vi "Register gRPC Methods.vi"(8 "error in (no error)":errorcluster, 11 "Template Server in":refnum<class "HVC9.lvclass">) -> (0 "error out":errorcluster, 3 "Template Server out":refnum<class "HVC9.lvclass">)   [LabVIEW 2019, in "HVC9.lvlib" / "HVC9.lvclass"]
uses:
  HVC9.lvclass
  typeDefs/Server Internal UEs.ctl
  typeDefs/Server Internal Message.ctl
  typeDefs/Server gRPC UEs.ctl
  gRPC lvSupport/Server API/typeDefs/gRPCId Cluster.ctl
  gRPC lvSupport/Server API/typeDefs/grpcId.ctl
  HVC9.lvclass/HVC9.ctl
  gRPC lvSupport/gprc-lvsupport.lvlib
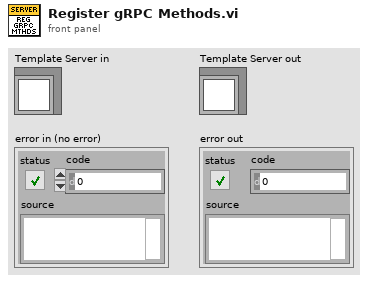
[diagram p1: front panel]
types:
  T1 = typedef "HVC9.lvlib/HVC9.lvclass/Server gRPC UEs.ctl" = cluster{"Invoke gRPC UE":refnum<user-event>, "Query gRPC UE":refnum<user-event>, "Register gRPC UE":refnum<user-event>, "OpenNI2564ASession gRPC UE":refnum<user-event>, "CloseNI2564AChannel gRPC UE":refnum<user-event>, "OpenNI2564AChannel gRPC UE":refnum<user-event>, "DisconnectAllNI2564AChannels gRPC UE":refnum<user-event>, "CloseNI2564ASession gRPC UE":refnum<user-event>, "ResetNI2564A gRPC UE":refnum<user-event>, "OpenNI2564BSession gRPC UE":refnum<user-event>, "CloseNI2564BChannel gRPC UE":refnum<user-event>, "OpenNI2564BChannel gRPC UE":refnum<user-event>, "DisconnectAllNI2564BChannels gRPC UE":refnum<user-event>, "CloseNI2564BSession gRPC UE":refnum<user-event>, "ResetNI2564B gRPC UE":refnum<user-event>}
  T2 = typedef "HVC9.lvlib/HVC9.lvclass/Server Internal UEs.ctl" = cluster{"Invoke Internal UE":refnum<user-event>, "Query Internal UE":refnum<user-event>, "Register Internal UE":refnum<user-event>, "OpenNI2564ASession Internal UE":refnum<user-event>, "CloseNI2564AChannel Internal UE":refnum<user-event>, "OpenNI2564AChannel Internal UE":refnum<user-event>, "DisconnectAllNI2564AChannels Internal UE":refnum<user-event>, "CloseNI2564ASession Internal UE":refnum<user-event>, "ResetNI2564A Internal UE":refnum<user-event>, "OpenNI2564BSession Internal UE":refnum<user-event>, "CloseNI2564BChannel Internal UE":refnum<user-event>, "OpenNI2564BChannel Internal UE":refnum<user-event>, "DisconnectAllNI2564BChannels Internal UE":refnum<user-event>, "CloseNI2564BSession Internal UE":refnum<user-event>, "ResetNI2564B Internal UE":refnum<user-event>}
  T3 = typedef "HVC9.lvlib/gprc-lvsupport.lvlib/grpcId.ctl" = u64
  T4 = typedef "HVC9.lvlib/HVC9.lvclass/Server Internal Message UE.ctl" = refnum<user-event>
  T5 = typedef "HVC9.lvlib/gprc-lvsupport.lvlib/gRPCId Cluster UE.ctl" = refnum<user-event>
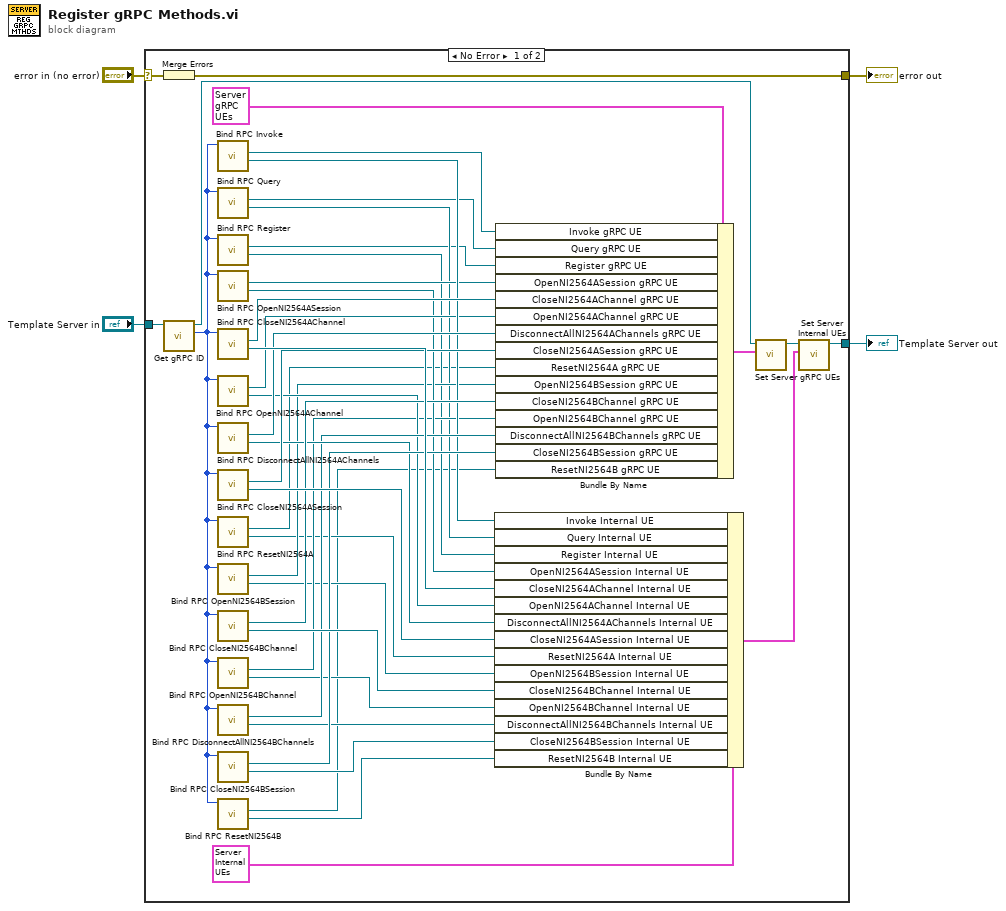
[diagram p0: block diagram]
diagram:
  n1 = case shown="No Error" "error in (no error)" {
    selector: "error in (no error)" -> [w36 w46]
    tunnel: "Template Server in" -> [w44 w47]
    tunnel: [w43 w46] -> w3
    tunnel: [w42 w47] -> w2
    frame No Error {
      n2 = Merge Errors(w36) -> (w43:errorcluster)
      n3 = call "Get gRPC ID.vi"("OOP Server in"=w44) -> ("gRPC ID"=w35:T3, "OOP Server out"=w45:refnum<class "HVC9.lvclass">)  [unwired: 9 in]
      n4 = call "Bind RPC Invoke.vi"("gRPCid server in"=w35) -> ("Invoke Internal UE"=w22:T4, "Invoke gRPC UE"=w21:T5)  [unwired: 7 in, 2 out]
      n5 = call "Bind RPC Query.vi"("gRPCid server in"=w35) -> ("Query Internal UE"=w12:T4, "Query gRPC UE"=w11:T5)  [unwired: 7 in, 2 out]
      n6 = call "Bind RPC Register.vi"("gRPCid server in"=w35) -> ("Register Internal UE"=w10:T4, "Register gRPC UE"=w9:T5)  [unwired: 7 in, 2 out]
      n7 = call "Bind RPC OpenNI2564ASession.vi"("gRPCid server in"=w35) -> ("OpenNI2564ASession Internal UE"=w18:T4, "OpenNI2564ASession gRPC UE"=w17:T5)  [unwired: 7 in, 2 out]
      n8 = call "Bind RPC CloseNI2564AChannel.vi"("gRPCid server in"=w35) -> ("CloseNI2564AChannel Internal UE"=w34:T4, "CloseNI2564AChannel gRPC UE"=w33:T5)  [unwired: 7 in, 2 out]
      n9 = call "Bind RPC OpenNI2564AChannel.vi"("gRPCid server in"=w35) -> ("OpenNI2564AChannel Internal UE"=w20:T4, "OpenNI2564AChannel gRPC UE"=w19:T5)  [unwired: 7 in, 2 out]
      n10 = call "Bind RPC DisconnectAllNI2564AChannels.vi"("gRPCid server in"=w35) -> ("DisconnectAllNI2564AChannels Internal UE"=w26:T4, "DisconnectAllNI2564AChannels gRPC UE"=w25:T5)  [unwired: 7 in, 2 out]
      n11 = call "Bind RPC CloseNI2564ASession.vi"("gRPCid server in"=w35) -> ("CloseNI2564ASession Internal UE"=w32:T4, "CloseNI2564ASession gRPC UE"=w31:T5)  [unwired: 7 in, 2 out]
      n12 = call "Bind RPC ResetNI2564A.vi"("gRPCid server in"=w35) -> ("ResetNI2564A Internal UE"=w8:T4, "ResetNI2564A gRPC UE"=w7:T5)  [unwired: 7 in, 2 out]
      n13 = call "Bind RPC OpenNI2564BSession.vi"("gRPCid server in"=w35) -> ("OpenNI2564BSession Internal UE"=w14:T4, "OpenNI2564BSession gRPC UE"=w13:T5)  [unwired: 7 in, 2 out]
      n14 = call "Bind RPC CloseNI2564BChannel.vi"("gRPCid server in"=w35) -> ("CloseNI2564BChannel Internal UE"=w30:T4, "CloseNI2564BChannel gRPC UE"=w29:T5)  [unwired: 7 in, 2 out]
      n15 = call "Bind RPC OpenNI2564BChannel.vi"("gRPCid server in"=w35) -> ("OpenNI2564BChannel Internal UE"=w16:T4, "OpenNI2564BChannel gRPC UE"=w15:T5)  [unwired: 7 in, 2 out]
      n16 = call "Bind RPC DisconnectAllNI2564BChannels.vi"("gRPCid server in"=w35) -> ("DisconnectAllNI2564BChannels Internal UE"=w24:T4, "DisconnectAllNI2564BChannels gRPC UE"=w23:T5)  [unwired: 7 in, 2 out]
      n17 = call "Bind RPC CloseNI2564BSession.vi"("gRPCid server in"=w35) -> ("CloseNI2564BSession Internal UE"=w28:T4, "CloseNI2564BSession gRPC UE"=w27:T5)  [unwired: 7 in, 2 out]
      n18 = call "Bind RPC ResetNI2564B.vi"("gRPCid server in"=w35) -> ("ResetNI2564B Internal UE"=w6:T4, "ResetNI2564B gRPC UE"=w5:T5)  [unwired: 7 in, 2 out]
      n19 = Bundle By Name ("Bundle Internal UEs")(cluster=T2 {"Invoke Internal UE"=refnum, "Query Internal UE"=refnum, "Register Internal UE"=refnum, "OpenNI2564ASession Internal UE"=refnum, "CloseNI2564AChannel Internal UE"=refnum, "OpenNI2564AChannel Internal UE"=refnum, "DisconnectAllNI2564AChannels Internal UE"=refnum, "CloseNI2564ASession Internal UE"=refnum, "ResetNI2564A Internal UE"=refnum, "OpenNI2564BSession Internal UE"=refnum, "CloseNI2564BChannel Internal UE"=refnum, "OpenNI2564BChannel Internal UE"=refnum, "DisconnectAllNI2564BChannels Internal UE"=refnum, "CloseNI2564BSession Internal UE"=refnum, "ResetNI2564B Internal UE"=refnum} ("Server Internal UEs"), "Invoke Internal UE"=w22, "Query Internal UE"=w12, "Register Internal UE"=w10, "OpenNI2564ASession Internal UE"=w18, "CloseNI2564AChannel Internal UE"=w34, "OpenNI2564AChannel Internal UE"=w20, "DisconnectAllNI2564AChannels Internal UE"=w26, "CloseNI2564ASession Internal UE"=w32, "ResetNI2564A Internal UE"=w8, "OpenNI2564BSession Internal UE"=w14, "CloseNI2564BChannel Internal UE"=w30, "OpenNI2564BChannel Internal UE"=w16, "DisconnectAllNI2564BChannels Internal UE"=w24, "CloseNI2564BSession Internal UE"=w28, "ResetNI2564B Internal UE"=w6) -> (w41:T2)
      n20 = Bundle By Name ("Bundle gRPC UEs")(cluster=T1 {"Invoke gRPC UE"=refnum, "Query gRPC UE"=refnum, "Register gRPC UE"=refnum, "OpenNI2564ASession gRPC UE"=refnum, "CloseNI2564AChannel gRPC UE"=refnum, "OpenNI2564AChannel gRPC UE"=refnum, "DisconnectAllNI2564AChannels gRPC UE"=refnum, "CloseNI2564ASession gRPC UE"=refnum, "ResetNI2564A gRPC UE"=refnum, "OpenNI2564BSession gRPC UE"=refnum, "CloseNI2564BChannel gRPC UE"=refnum, "OpenNI2564BChannel gRPC UE"=refnum, "DisconnectAllNI2564BChannels gRPC UE"=refnum, "CloseNI2564BSession gRPC UE"=refnum, "ResetNI2564B gRPC UE"=refnum} ("gRPC Server Method Events"), "Invoke gRPC UE"=w21, "Query gRPC UE"=w11, "Register gRPC UE"=w9, "OpenNI2564ASession gRPC UE"=w17, "CloseNI2564AChannel gRPC UE"=w33, "OpenNI2564AChannel gRPC UE"=w19, "DisconnectAllNI2564AChannels gRPC UE"=w25, "CloseNI2564ASession gRPC UE"=w31, "ResetNI2564A gRPC UE"=w7, "OpenNI2564BSession gRPC UE"=w13, "CloseNI2564BChannel gRPC UE"=w29, "OpenNI2564BChannel gRPC UE"=w15, "DisconnectAllNI2564BChannels gRPC UE"=w23, "CloseNI2564BSession gRPC UE"=w27, "ResetNI2564B gRPC UE"=w5) -> (w38:T1)
      n21 = call "Set Server gRPC UEs.vi"("Server gRPC UEs"=w38, "OOP Server in"=w45) -> ("OOP Server out"=w39:refnum<class "HVC9.lvclass">)  [unwired: 9 in]
      n22 = call "Set Server Internal UEs.vi"("Server Internal UEs"=w41, "OOP Server in"=w39) -> ("OOP Server out"=w42:refnum<class "HVC9.lvclass">)  [unwired: 9 in]
    }
    frame Error {
    }
  }
  "error out" <- w3
  "Template Server out" <- w2
